vi "DOutTest.vi"() -> ()   [LabVIEW 2018]
uses:
  <vilib>/express/express shared/transition.llb/Dynamic To Waveform Array.vi
  <vilib>/express/express signal manip/GetorSetDDTAttributes/Set DDT Attributes/SetT0.vi
  <vilib>/express/express signal manip/GetorSetDDTAttributes/Set DDT Attributes/sub Set StartTimeStamp.vi
  <vilib>/express/express shared/transition.llb/Waveform Array To Dynamic.vi
  <vilib>/express/express signal manip/GetorSetDDTAttributes/Set DDT Attributes/Set DDT Properties.xnode
  <vilib>/express/express signal manip/GetorSetDDTAttributes/Set DDT Attributes/Set DDT Attributes.lvlib
panel:
  in  "Valve Log Name":string="Log_Valves"
  in  "Load Cell Log Name":string="Log_LoadCell"
  in  "Sensor Log Name":string="Log_Sensors"
  in  "Log Folder":path=path "C:/LPLDocs"
  out "Sensor Readings":dbl[](array[numeric]) format="%#_13g"
  in  "System State":u16(ring) items=["Testing", "Safe", "Armed", "Pressurized", "Firing", "Aborted", "Fire Complete"]
  in  "Record":bool
  in  "Pump":bool
  in  "Ignition":bool
  in  "Ignition Type":u16(ring)=2 items=["Spark Plug", "Glow Plug", "Pyro"]
  out "NC-OP Status":bool
  out "NC-FP Status":bool
  out "NC-OI Status":bool
  out "NC-O Status":bool
  out "NC-P Status":bool
  out "NC-FI Status":bool
  out "NC-F Status":bool
  out "NO-P Status":bool
  in  "NC-OP":bool
  in  "NC-FP":bool
  in  "NC-OI":bool
  in  "NC-O":bool
  in  "NC-F":bool
  in  "NC-P":bool
  in  "NO-P":bool
  in  "NC-FI":bool
  # "PT-1P"
  # "DOut Unit Test Procedures:\n\nReturn to default position after each test.\n\nSetup:\nPressurize the compressed air tank\nAttach a pressure source to the pressurant line (this may be the air compressor)\nPower on the DAQ box, hook up the leads to the battery within the box\nVerify all wire leads to the fuel pump, igniter, valves, and PT-1P\n\n1) Actuate each individual valve on, then off.\n        Verify visually that each ball valve turns to the correct position when actuated.\n        Verify using a magnetometer that each solenoid activates when actuated.\n2) Actuate all valves so they are all on at once.\n        Verify visually and using a magnetometer that all valves are open except NO-P, which should be closed.\n3) Set the Ignition Type to Pyro and activate Ignition (ensure no pyro ignitor is attached, first!)\n        Verify using a multimeter that the ignitor leads read +/-12V.\n        Deactivate Ignition and verify that the leads read 0V\n4) Activate the pump (ensure there is fluid in the tank to be be pumped)\n        Verify audially that the fuel pump activates\n5) Check the Sensor Readings UI element and add pressure upstream of NC-P\n        Verify that voltage readings are nonzero\n6) Set the Ignition Type to Spark Plug and actuate NC-IO and NC-IF\n        Verify that neither solenoid has actuated\n7) Set the Ignition Type to Spark Plug and attach an oscilliscope to the ignitor leads\n        Verify that the oscilliscope wave is flat\n        Activate Ignition\n        Verify that the oscilliscope reads a stable waveform with a duty cycle of ~30%\n8) Attach the spark plug and ignition coil to the ignition leads. Tape the ground lead to the spark plug body.\n        Set Ignition Type to Spark Plug and activate Ignition\n        Verify that sparks arc across the head of the spark plug.\n9) Activate Record and run tests 1, 3, 4, and 8. The tests may be performed in any order and Record may be\ndeactivated between each test. Open the log file corresponding to this run located at C:/LPLDocs\n        Verify that time data appears in the X column and is accurate to the span of the tests\n        Test 1: Verify that the numbers 1, 2, 4, 8, 16, 32, 64, 128 appear under the Valves column when  NC-P, \nNO-P, NC-F, NC-FI, NC-FP, NC-O, NC-OI, NC-OP are actuated, respectively\n        Test 3: Verify that 1 appears under the Igniter column when Ignition is activated\n        Test 4: Verify that 1 appears under the Pump column when Pump is activated\n        Test 7: Verify that 1 appears under the Igniter column when Ignition is activated, and that the value is\nconstant (ie not a waveform like the electrical signal)\n        Set System State to each possible value while recording, in sequence\n        Verify that  the states 0, 1, 2, 3, 4, 5, 6 appear in the System State column at the appropriate times\n        Verify the column for PT-1P is populated with accurate data."
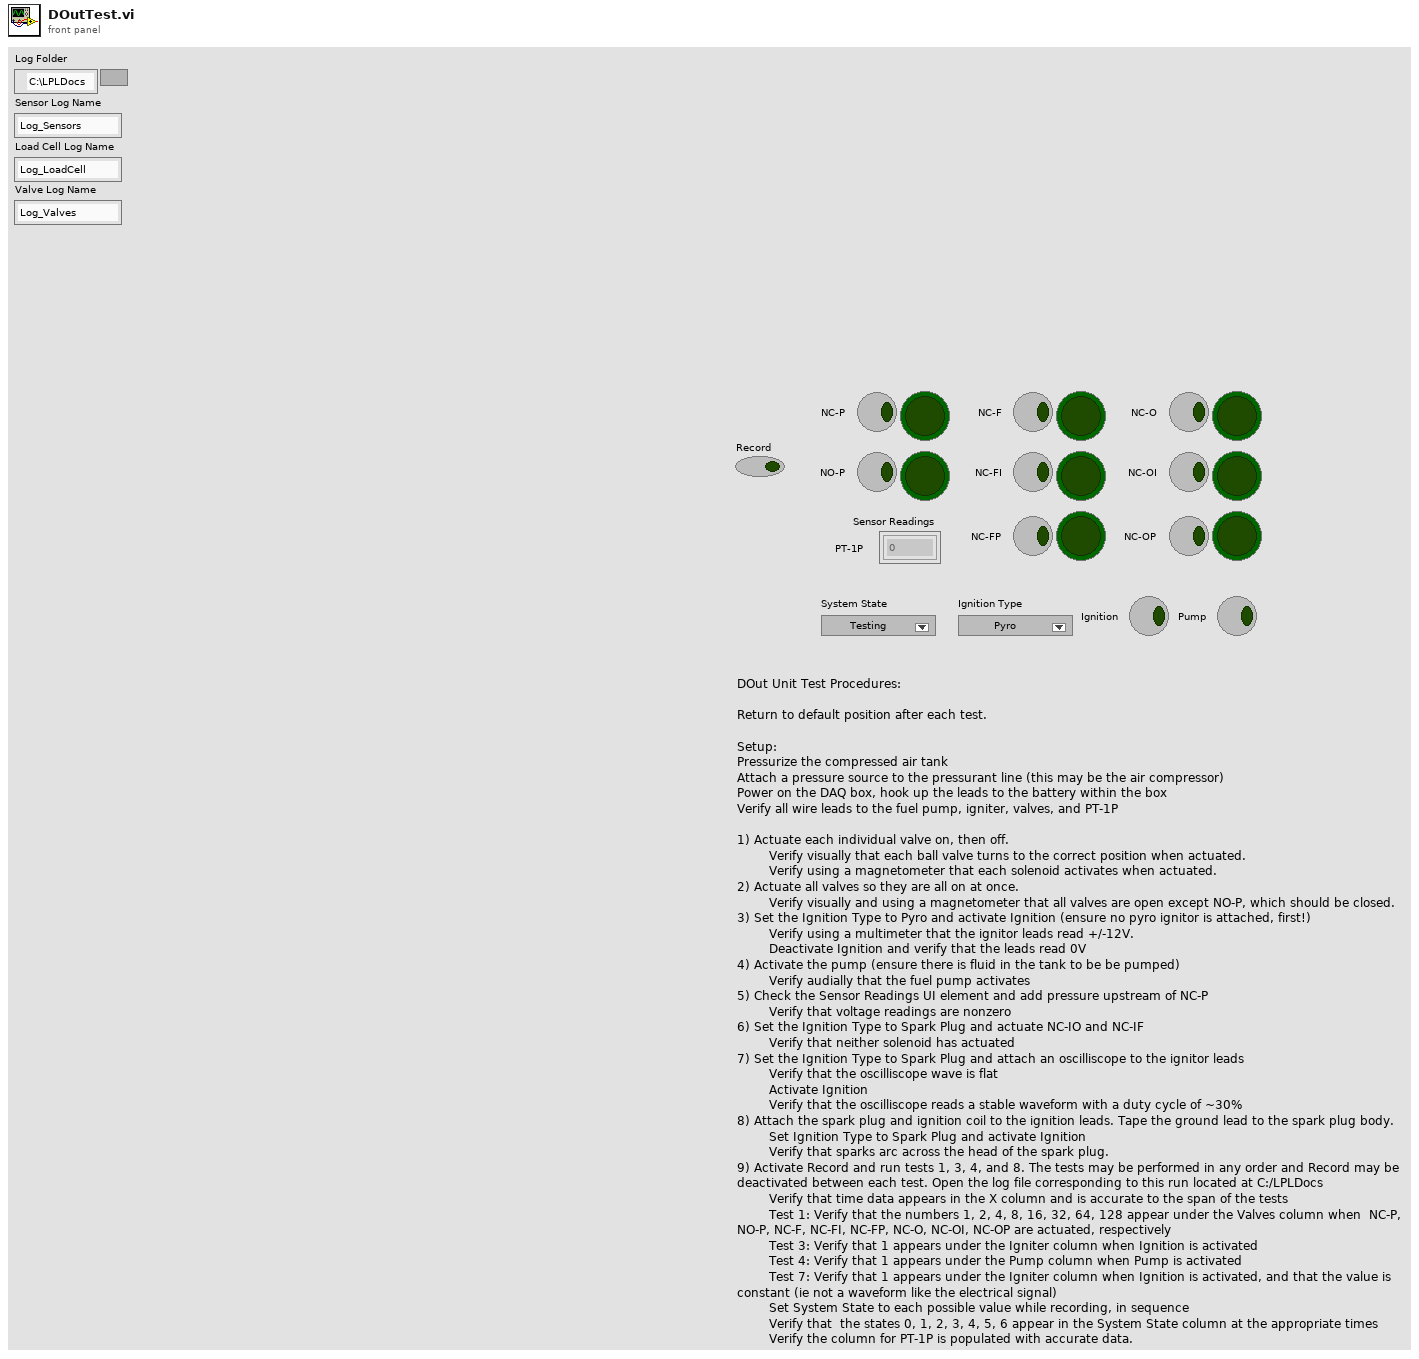
[diagram p1: front panel]
types:
  T1 = enum16{"Normal", "Overdrive", "Ready for Overdrive End", "Ready for new file", "New file"}
  T2 = cluster{"SensorPath":path, "LoadCellPath":path, "ValvePath":path}
  T3 = cluster{"LoadCell Queue":refnum<queue>, "Sensor Queue":refnum<queue>, "Valve Queue":refnum<queue>}
  T4 = cluster{"Sensors":refnum<notifier>, "LoadCell":refnum<notifier>, "Fileout":refnum<notifier>, "UI":refnum<notifier>}
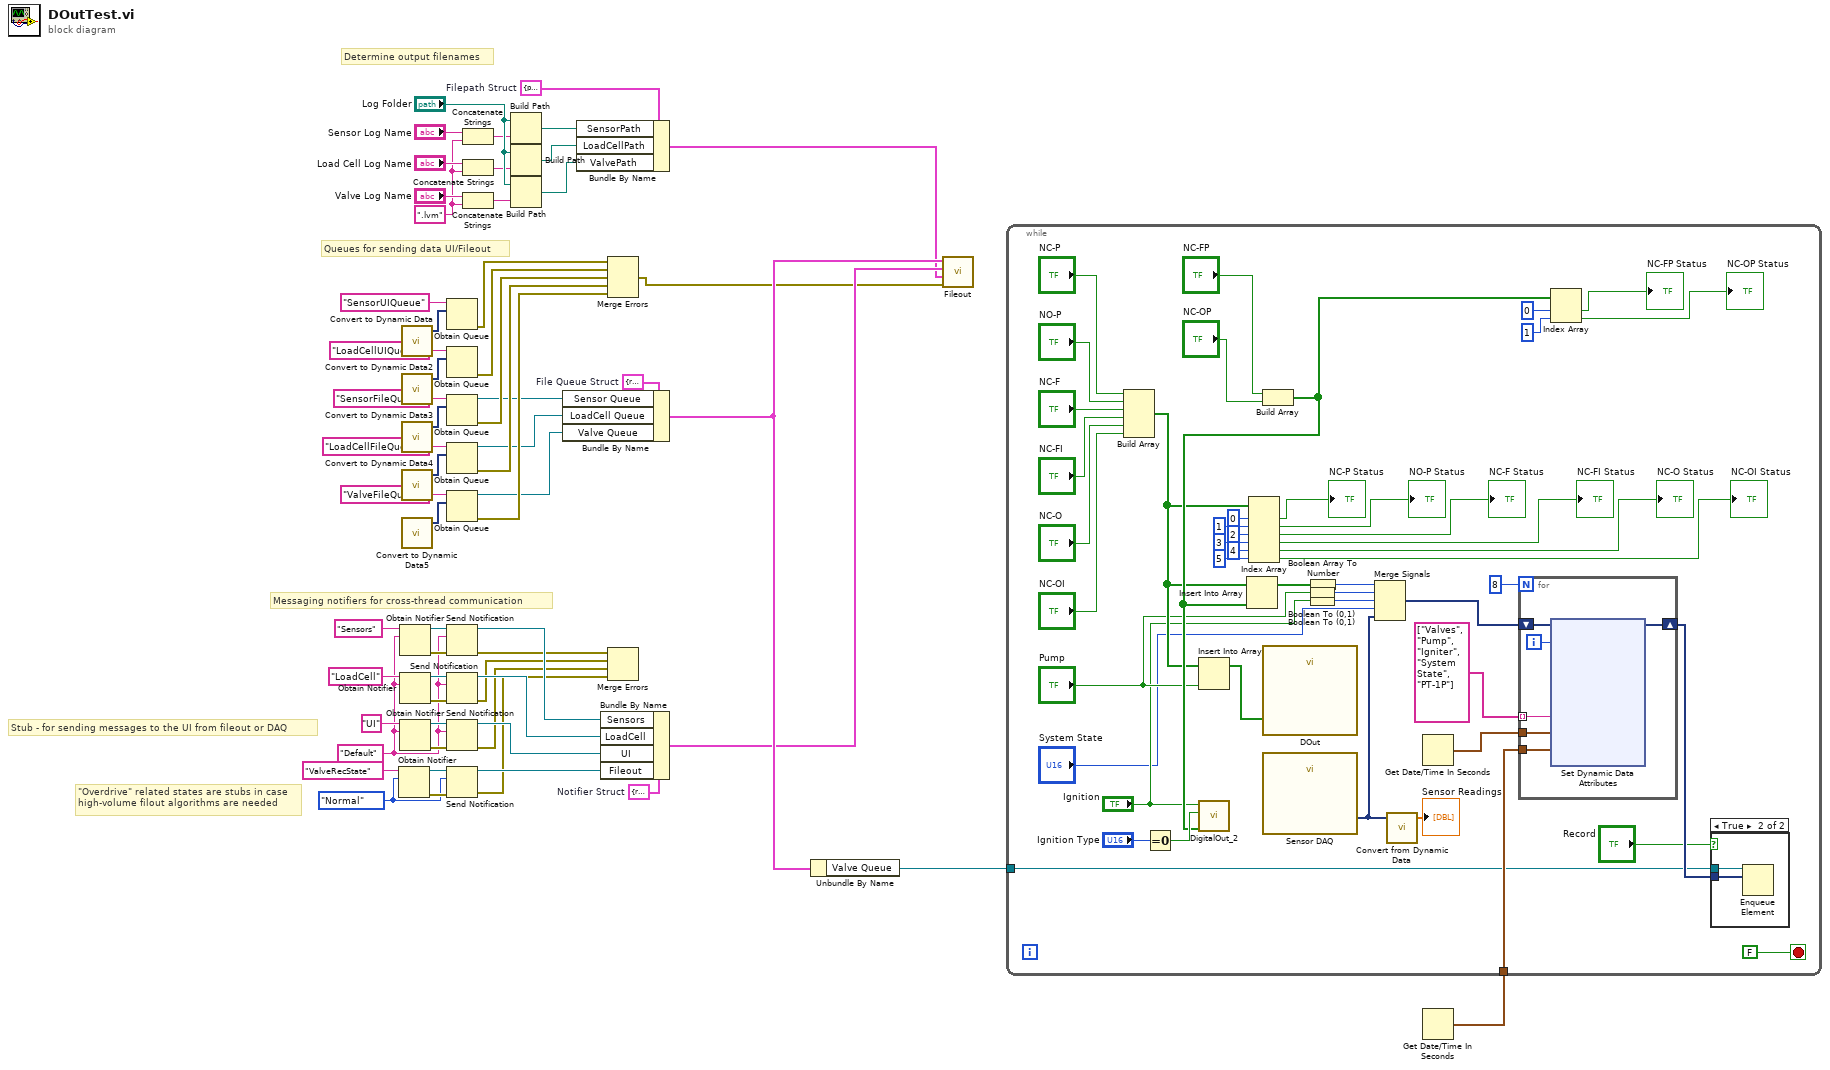
[diagram p0: block diagram]
diagram:
  w14 = ".lvm"
  w22 = T1."Normal" ("RecState")
  w13 = T2 {"SensorPath"=path "", "LoadCellPath"=path "", "ValvePath"=path ""}  # Filepath Struct
  w9 = T3 {"LoadCell Queue"=refnum, "Sensor Queue"=refnum, "Valve Queue"=refnum}  # File Queue Struct
  w27 = T4 {"Sensors"=refnum, "LoadCell"=refnum, "Fileout"=refnum, "UI"=refnum}  # Notifier Struct
  w26 = "Default" ("RecState")
  # "Messaging notifiers for cross-thread communication"
  # "Queues for sending data UI/Fileout"
  # "Determine output filenames"
  # "Stub - for sending messages to the UI from fileout or DAQ"
  # "\"Overdrive\" related states are stubs in case\nhigh-volume filout algorithms are needed"
  n1 = Obtain Notifier(name (unnamed)="ValveRecState", notification data type=w22) -> (notifier out=w24:refnum<notifier>, error out=w23:errorcluster)  [unwired: 2 in, 1 out]
  n2 = Obtain Notifier(name (unnamed)="Sensors", notification data type=w26) -> (notifier out=w52:refnum<notifier>, error out=w51:errorcluster)  [unwired: 2 in, 1 out]
  n3 = Obtain Notifier(name (unnamed)="LoadCell", notification data type=w26) -> (notifier out=w54:refnum<notifier>, error out=w55:errorcluster)  [unwired: 2 in, 1 out]
  n4 = Obtain Notifier(name (unnamed)="UI", notification data type=w26) -> (notifier out=w56:refnum<notifier>, error out=w57:errorcluster)  [unwired: 2 in, 1 out]
  n5 = call "Convert to Dynamic Data"() -> ("Dynamic Data Type"=w41:dynamicdata)  [unwired: 4 in]
  n6 = call "Convert to Dynamic Data2"() -> ("Dynamic Data Type"=w39:dynamicdata)  [unwired: 4 in]
  n7 = call "Convert to Dynamic Data3"() -> ("Dynamic Data Type"=w37:dynamicdata)  [unwired: 4 in]
  n8 = call "Convert to Dynamic Data4"() -> ("Dynamic Data Type"=w35:dynamicdata)  [unwired: 4 in]
  n9 = call "Convert to Dynamic Data5"() -> ("Dynamic Data Type"=w33:dynamicdata)  [unwired: 4 in]
  n10 = Obtain Queue(name (unnamed)="SensorUIQueue", element data type=w41) -> (error out=w32:errorcluster)  [unwired: 3 in, 2 out]
  n11 = Obtain Queue(name (unnamed)="LoadCellUIQueue", element data type=w39) -> (error out=w31:errorcluster)  [unwired: 3 in, 2 out]
  n12 = Obtain Queue(name (unnamed)="SensorFileQueue", element data type=w37) -> (queue out=w8:refnum<queue>, error out=w30:errorcluster)  [unwired: 3 in, 1 out]
  n13 = Obtain Queue(name (unnamed)="LoadCellFileQueue", element data type=w35) -> (queue out=w7:refnum<queue>, error out=w29:errorcluster)  [unwired: 3 in, 1 out]
  n14 = Obtain Queue(name (unnamed)="ValveFileQueue", element data type=w33) -> (queue out=w6:refnum<queue>, error out=w28:errorcluster)  [unwired: 3 in, 1 out]
  n15 = Send Notification(notification=w26, notifier=w52, error in (no error)=w51) -> (notifier out=w49:refnum<notifier>, error out=w45:errorcluster)
  n16 = Send Notification(notification=w26, notifier=w54, error in (no error)=w55) -> (notifier out=w48:refnum<notifier>, error out=w44:errorcluster)
  n17 = Send Notification(notification=w26, notifier=w56, error in (no error)=w57) -> (notifier out=w47:refnum<notifier>, error out=w43:errorcluster)
  n18 = Send Notification(notification=w22, notifier=w24, error in (no error)=w23) -> (notifier out=w50:refnum<notifier>, error out=w46:errorcluster)
  n19 = Concatenate Strings("Sensor Log Name", w14) -> (w17:string)
  n20 = Concatenate Strings("Load Cell Log Name", w14) -> (w16:string)
  n21 = Concatenate Strings("Valve Log Name", w14) -> (w15:string)
  n22 = Build Path(base path="Log Folder", name or relative path=w17) -> (appended path=w12:path)
  n23 = Build Path(base path="Log Folder", name or relative path=w16) -> (appended path=w11:path)
  n24 = Build Path(base path="Log Folder", name or relative path=w15) -> (appended path=w10:path)
  n25 = Bundle By Name(cluster=w9, "Sensor Queue"=w8, "LoadCell Queue"=w7, "Valve Queue"=w6) -> (w5:T3)
  n26 = Bundle By Name(cluster=w13, "SensorPath"=w12, "LoadCellPath"=w11, "ValvePath"=w10) -> (w2:T2)
  n27 = Bundle By Name(cluster=w27, "Sensors"=w49, "LoadCell"=w48, "UI"=w47, "Fileout"=w50) -> (w3:T4)
  n28 = Merge Errors(w32, w31, w30, w29, w28) -> (w1:errorcluster)
  n29 = Merge Errors(w45, w44, w43, w46) -> ()  [unwired: 1 out]
  n30 = Unbundle By Name(w5) -> ("Valve Queue"=w4:refnum<queue>)
  n31 = call "Fileout.vi"("error in (no error)"=w1, "Filepaths"=w2, "Message Notifiers"=w3, "File Queues"=w5) -> ()  [unwired: 7 in, 1 out]
  n32 = Get Date/Time In Seconds() -> (seconds since 1Jan1904=w60:timestamp)
  n33 = while {
    tunnel: w4 -> [w67]
    tunnel: w60 -> [w70]
    stop <- FALSE stop-if-true
    n34 = Build Array("NC-P", "NO-P", "NC-F", "NC-FI", "NC-O", "NC-OI") -> (w79:bool[])
    n35 = Equal To 0?(x="Ignition Type") -> (x = 0?=w81:bool)
    n36 = Insert Into Array(array=w79, new element="Pump") -> (w78:bool[])  [unwired: 1 in]
    n37 = Index Array(array=w79, index #1=0 ("index"), index #2=1 ("index"), index #3=2 ("index"), index #4=3 ("index"), index #5=4 ("index"), index #6=5 ("index")) -> (element #1=→"NC-P Status":bool, element #2=→"NO-P Status":bool, element #3=→"NC-F Status":bool, element #4=→"NC-FI Status":bool, element #5=→"NC-O Status":bool, element #6=→"NC-OI Status":bool)
    n38 = Build Array("NC-FP", "NC-OP") -> (w80:bool[])
    n39 = call "DigitalOut_2.vi"("Purge Valves"=w80, "Spark Arm"=w81, "Ignition!"="Ignition") -> ()  [unwired: 8 in, 1 out]
    n40 = Insert Into Array(array=w79, new element=w80) -> (w77:bool[])  [unwired: 1 in]
    n41 = call "DOut"("data"=w78) -> ()  [unwired: 17 in, 2 out]
    n42 = call "Sensor DAQ"() -> ("data"=w62:dynamicdata)  [unwired: 17 in, 2 out]
    n43 = Boolean To (0,1)(Boolean="Pump") -> (0, 1=w65:i16)
    n44 = Boolean To (0,1)(Boolean="Ignition") -> (0, 1=w64:i16)
    n45 = Boolean Array To Number(Boolean array=w77) -> (number=w74:u32)
    n46 = Merge Signals(w74, w65, w64, "System State", w62) -> (w72:dynamicdata)
    n47 = call "Convert from Dynamic Data"("Dynamic Data Type"=w62) -> ("Array"=→"Sensor Readings":dbl[])  [unwired: 3 in]
    n48 = Get Date/Time In Seconds() -> (seconds since 1Jan1904=w69:timestamp)
    n49 = for {
      N: 8 -> [_]
      tunnel: string[] ["Valves", "Pump", "Igniter", "System State", "PT-1P"] -> [w114] mode=indexing
      tunnel: w70 -> [w113]
      tunnel: w69 -> [w112]
      shift-right: [w111] -> w68
      shift-left: w72 -> [w115]
      i -> [w110]
      n50 = xnode "Set Dynamic Data Attributes"("Signal Name"=w114, "Start Timestamp"=w113, "Timestamp"=w112, "Signals In"=w115, "Signal Index"=w110) -> ("Signals Out"=w111:dynamicdata)  [unwired: 1 in, 1 out]
    }
    n51 = Index Array(array=w80, index #1=0 ("index"), index #2=1 ("index")) -> (element #1=→"NC-FP Status":bool, element #2=→"NC-OP Status":bool)
    n52 = case shown="True" "Record" {
      tunnel: w68 -> [_ w109]
      tunnel: w67 -> [_ w108]
      frame False {
      }
      frame True {
        n53 = Enqueue Element(queue=w108, element=w109) -> ()  [unwired: 2 in, 3 out]
      }
    }
  }
